vi "Untitled 5.vi"() -> ()   [LabVIEW 2019]
panel:
  in  "stop 3":bool
  in  "stop":bool
  out "x+y 2":i32
  out "x+y":i32
  in  "Boolean":bool
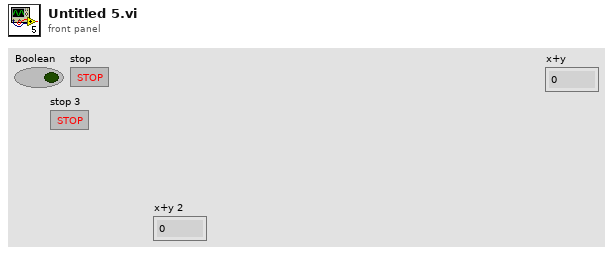
[diagram p1: front panel]
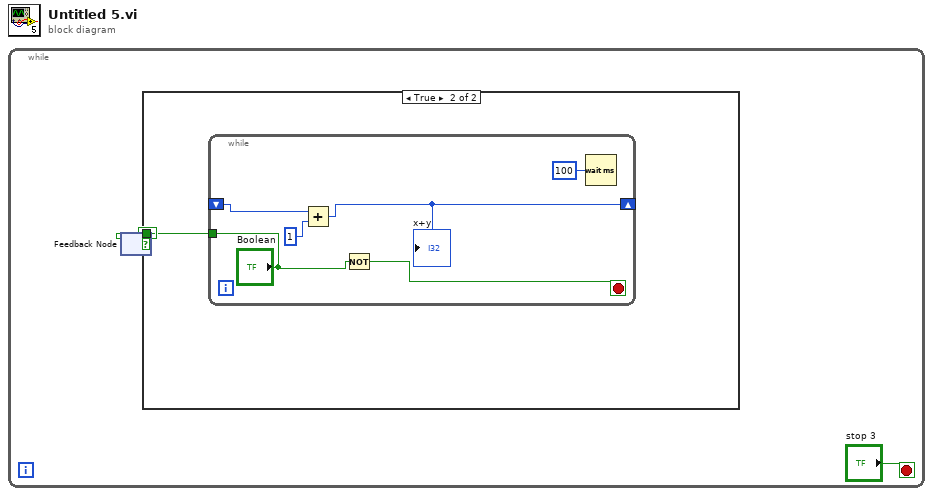
[diagram p0: block diagram]
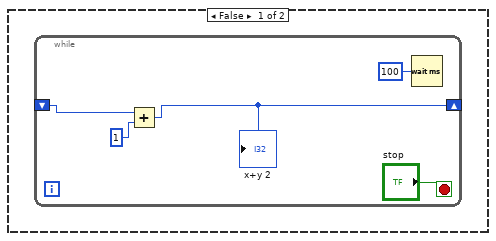
[diagram p2: hidden frame]
diagram:
  n1 = while {
    stop <- "stop 3" stop-if-true
    n2 = feedback #1() -> (w1:bool)  [unwired: 1 in]
    n3 = case shown="True" w1 {
      tunnel: [_ w9] -> w2
      frame False {
        n4 = while {
          shift-right: [w7] -> _
          shift-left: _ -> [w8]
          stop <- "stop" stop-if-true
          n5 = Add(x=w8, y=1) -> (x+y=w7:i32)
          "x+y 2" <- w7
          n6 = Wait (ms)(milliseconds to wait=u32 100) -> ()  [unwired: 1 out]
        }
      }
      frame True {
        n7 = while {
          shift-right: [w14] -> _
          shift-left: _ -> [w15]
          tunnel: ["Boolean"] -> w9
          stop <- w10 stop-if-true
          n8 = Add(x=w15, y=1) -> (x+y=w14:i32)
          "x+y" <- w14
          n9 = Not(x="Boolean") -> (.not. x?=w10:bool)
          n10 = Wait (ms)(milliseconds to wait=u32 100) -> ()  [unwired: 1 out]
        }
      }
    }
    n11 = feedback-in #1(w2) -> ()
  }
